vi "writeCSV(create_replace).vi"(7 "Header":string[](array[string]), 8 "error in (no error)":errorcluster, 9 "Array":dbl[][](array[numeric]), 10 "file path (use dialog)":path=path "C:/Users/RoboIme/git/sslview/Util/Farias2.csv", 11 "Utilities in":refnum<class "Utilities.lvclass">) -> (0 "error out":errorcluster, 3 "Utilities out":refnum<class "Utilities.lvclass">)   [LabVIEW 2020, in "Utilities.lvclass"]
uses:
  Utilities.lvclass
panel:
  out "refnum out":refnum<file>
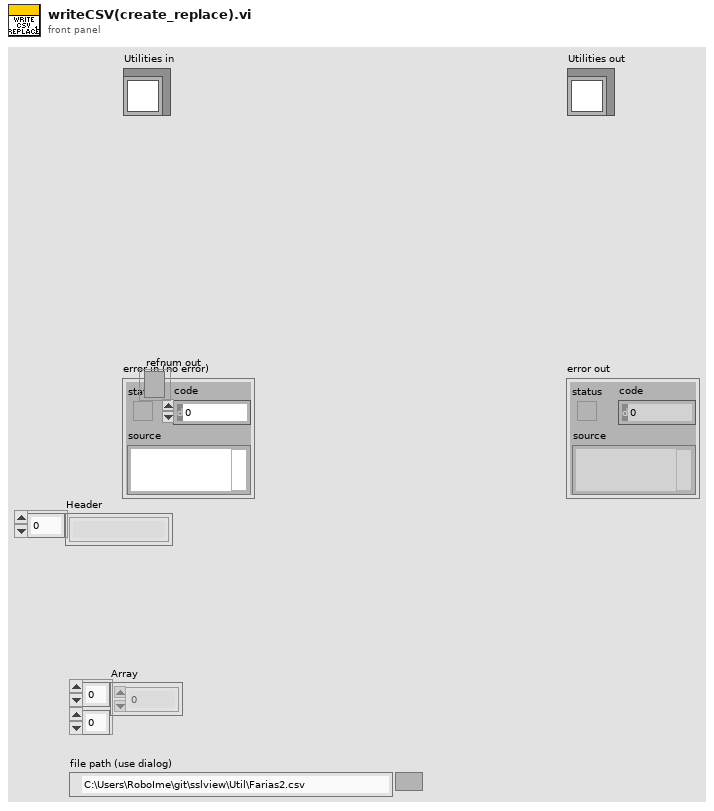
[diagram p1: front panel]
types:
  T1 = enum16{"open", "replace", "create", "open or create", "replace or create", "replace or create with confirmation"}
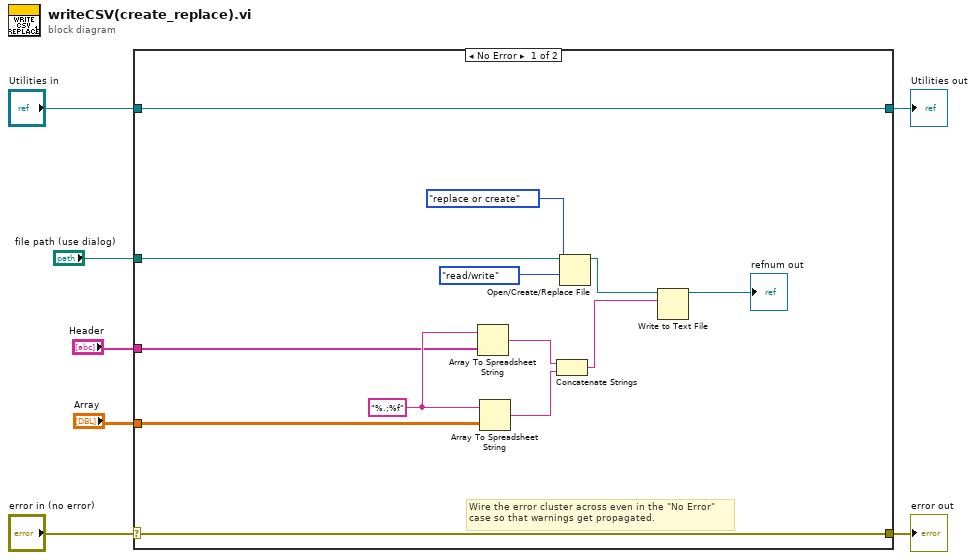
[diagram p0: block diagram]
diagram:
  n1 = case shown="No Error" "error in (no error)" {
    selector: "error in (no error)" -> [w19 w22]
    tunnel: [w19 w22] -> w6
    tunnel: [w20 w21] -> w4
    tunnel: "Utilities in" -> [w20 w21]
    tunnel: "file path (use dialog)" -> [w13 _]
    tunnel: "Array" -> [w18 _]
    tunnel: "Header" -> [w11 _]
    frame No Error {
      w12 = "%.;%f" ("format string")
      # "Wire the error cluster across even in the \"No Error\"\ncase so that warnings get propagated."
      n2 = Array To Spreadsheet String(array=w11, 3:w12) -> (spreadsheet string=w10:string)  [unwired: 1 in]
      n3 = Array To Spreadsheet String(array=w18, 3:w12) -> (spreadsheet string=w9:string)  [unwired: 1 in]
      n4 = Concatenate Strings(w10, w9) -> (w8:string)
      n5 = Open/Create/Replace File(file path (use dialog)=w13, operation (0:open)=T1."replace or create", access (0:read/write)=enum16{"read/write", "read-only", "write-only"}."read/write") -> (refnum out=w15:refnum<file>)  [unwired: 3 in, 2 out]
      n6 = Write to Text File(file (use dialog)=w15, text=w8) -> (refnum out=→"refnum out":refnum<file>)  [unwired: 2 in, 2 out]
    }
    frame Error {
    }
  }
  "error out" <- w6
  "Utilities out" <- w4
